vi "video.property_count.vi"(8 "error in":errorcluster, 11 "Video in":refnum<class "Video.lvclass">) -> (0 "error out":errorcluster, 3 "Video out":refnum<class "Video.lvclass">)   [LabVIEW 2020, in "Video.lvclass"]
doc: "Returns the number of properties on the video."
uses:
  Video.lvclass
  Video.lvclass/Video.ctl
  client.lvlib
panel:
  out "out_count out":u32
  in  "out_count":u32
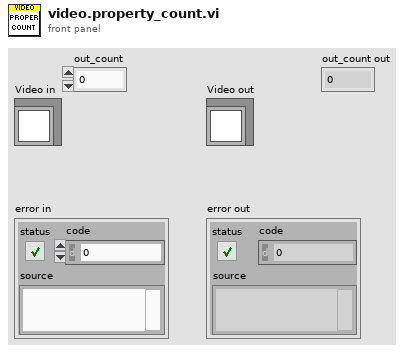
[diagram p1: front panel]
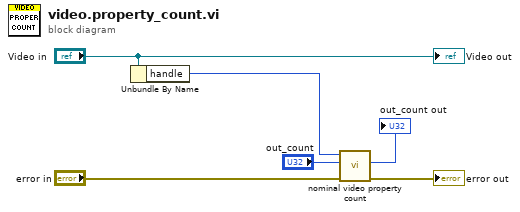
[diagram p0: block diagram]
diagram:
  n1 = Unbundle By Name("Video in") -> ("handle"=w4:i32)
  n2 = call "nominal video property count.vi"("error in (no error)"="error in", "out_count"="out_count", "video"=w4) -> ("error out"=→"error out":errorcluster, "out_count out"=→"out_count out":u32)  [unwired: 6 in, 1 out]
  "Video out" <- "Video in"
